vi "Calculate Normals for Mesh.vi"(9 "Color Binding Mode":T1(ring), 10 "Vertex Array":cluster{"X":sgl, "Y":sgl, "Z":sgl}[](array[cluster]), 11 "Draw Mode":T2(ring)) -> (3 "Normal Array":cluster{"X":sgl, "Y":sgl, "Z":sgl}[](array[cluster]))   [LabVIEW 2017, in "NI_3D Picture Control.lvlib"]
uses:
  <vilib>/picture/3D Picture Control/NI_3D Picture Control.lvlib
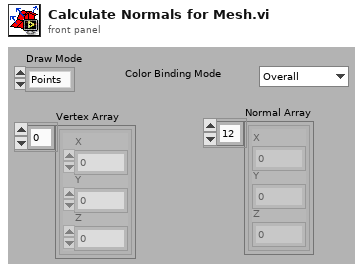
[diagram p1: front panel]
types:
  T1 = enum16{"Overall", "Per Primitive", "Per Vertex", "Binding Off"}
  T2 = enum16{"Points", "Lines", "Line Strip", "Line Loop", "Triangles", "Triangle Strip", "Triangle Fan", "Quads", "Quad Strip", "Polygon"}
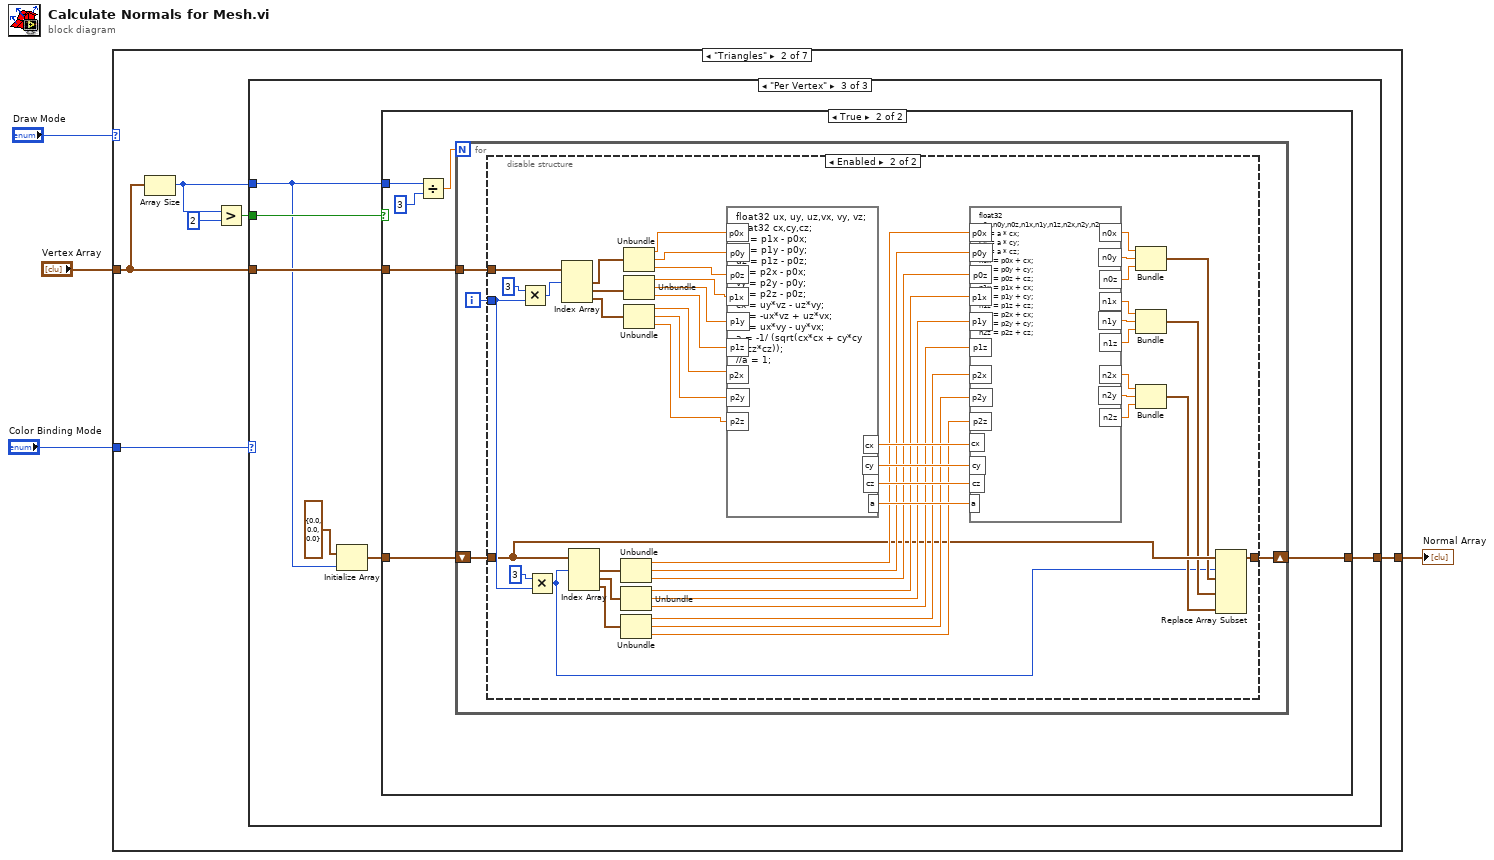
[diagram p0: block diagram]
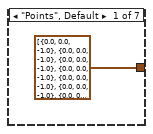
[diagram p2: hidden frame]
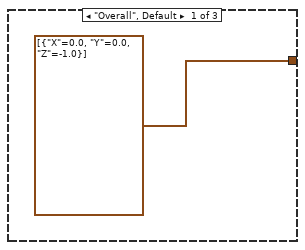
[diagram p3: hidden frame]
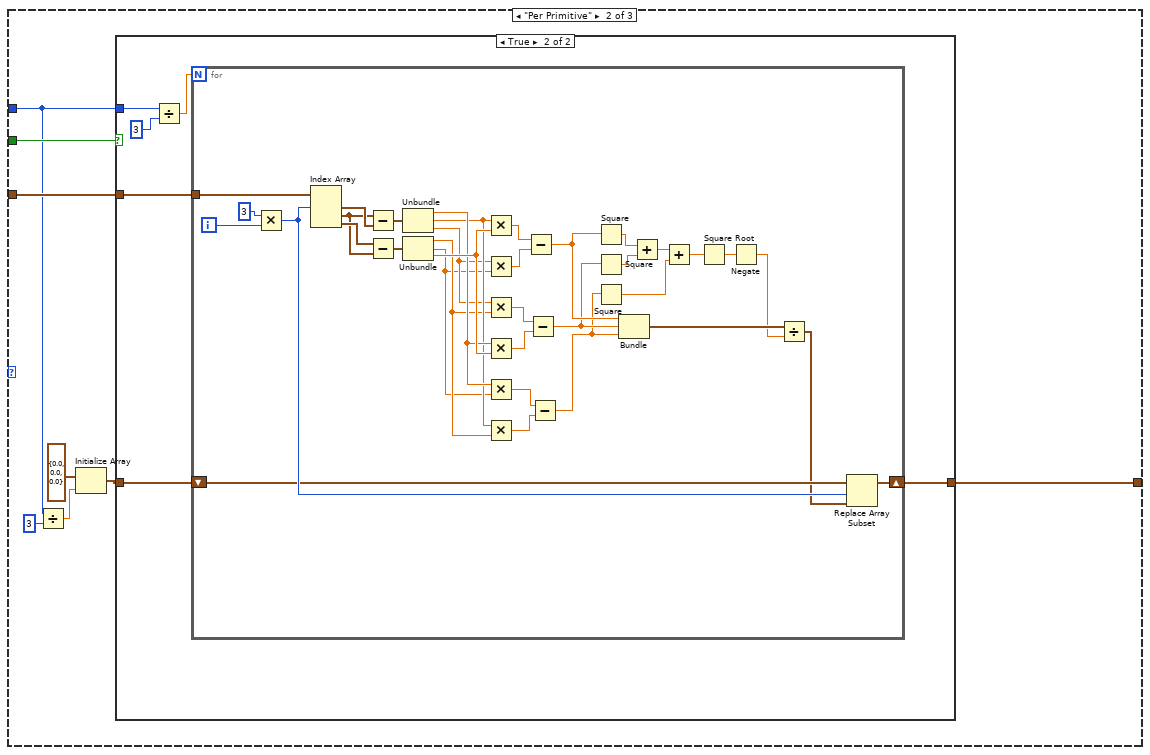
[diagram p4: hidden frame]
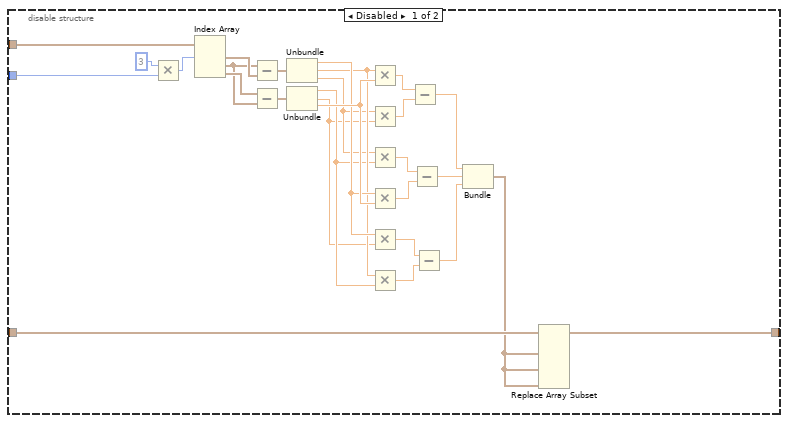
[diagram p7: hidden frame]
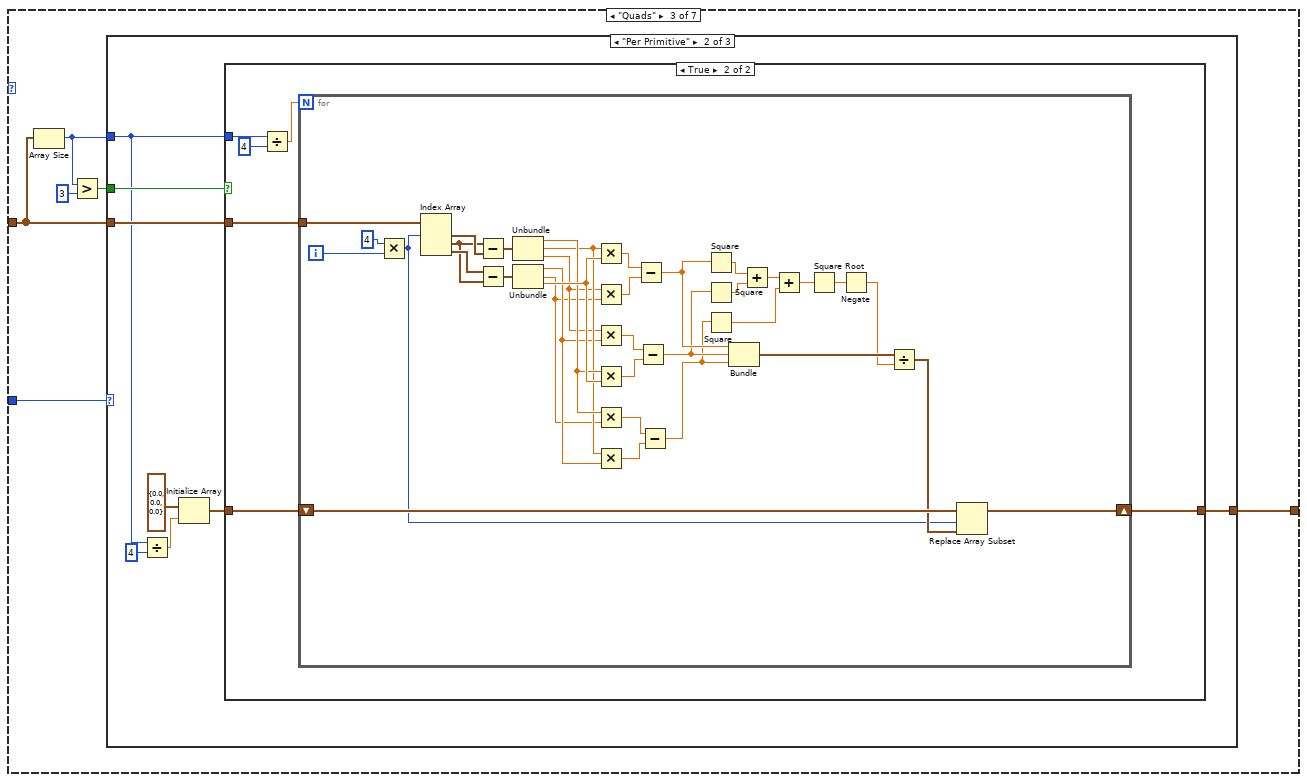
[diagram p8: hidden frame]
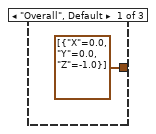
[diagram p9: hidden frame]
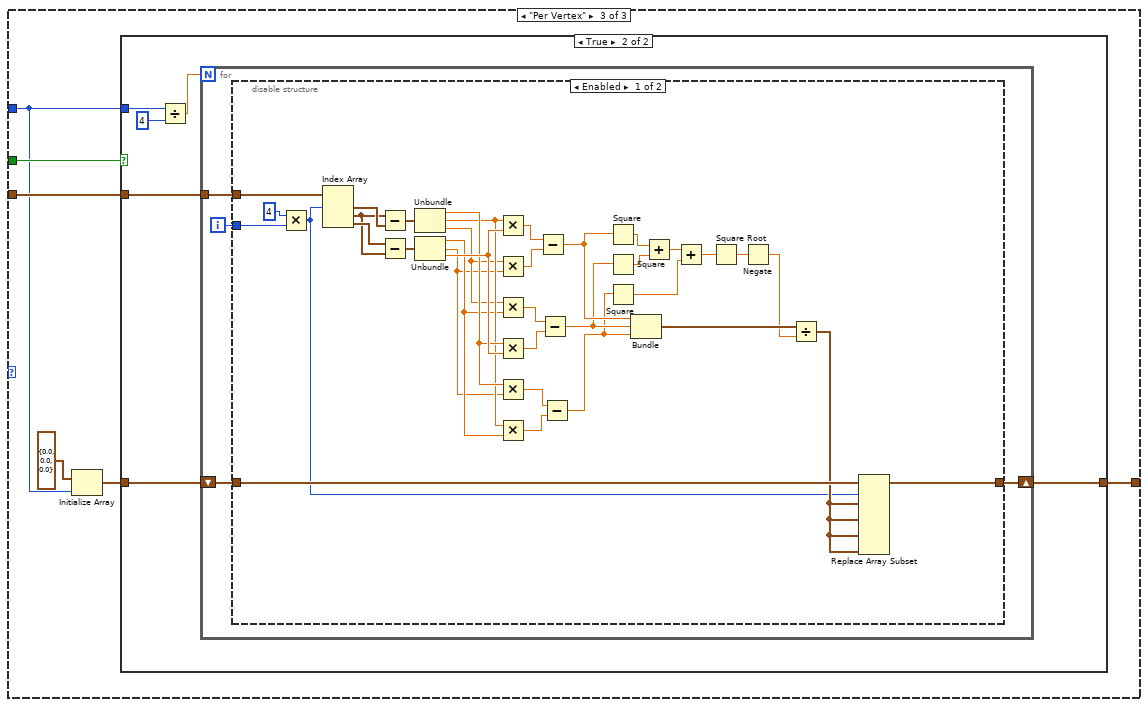
[diagram p11: hidden frame]
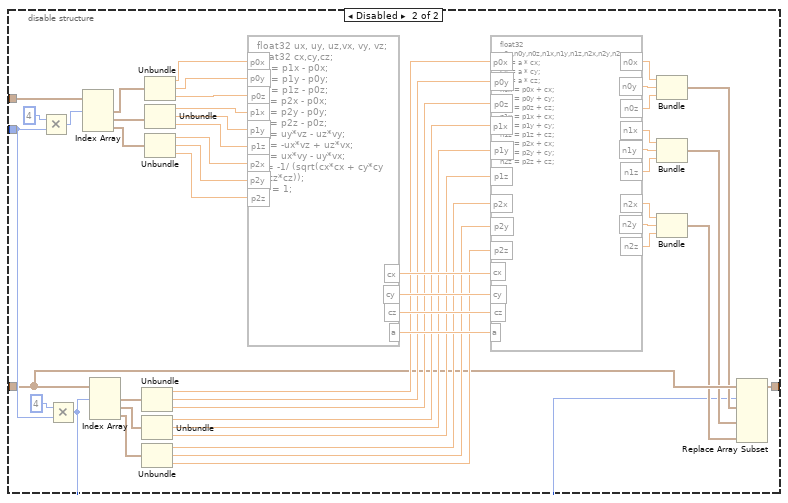
[diagram p13: hidden frame]
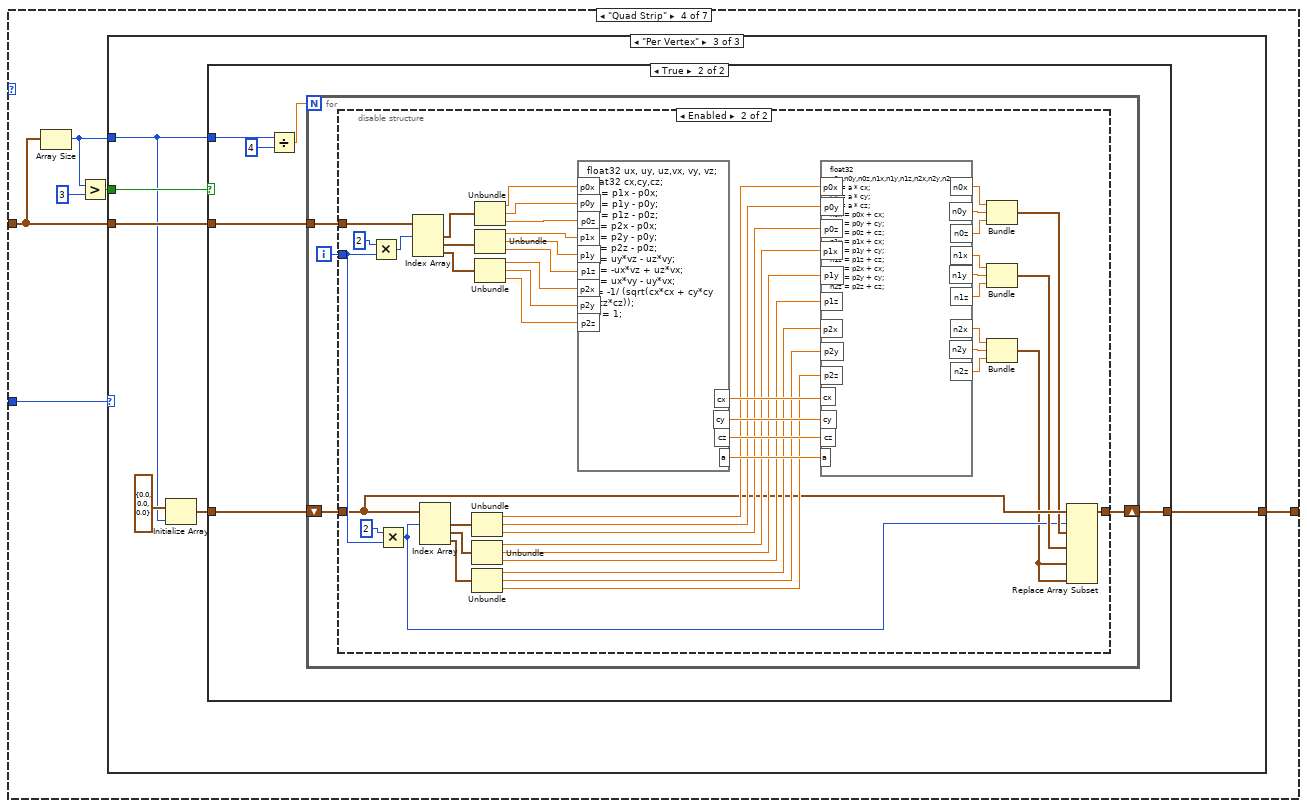
[diagram p14: hidden frame]
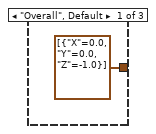
[diagram p15: hidden frame]
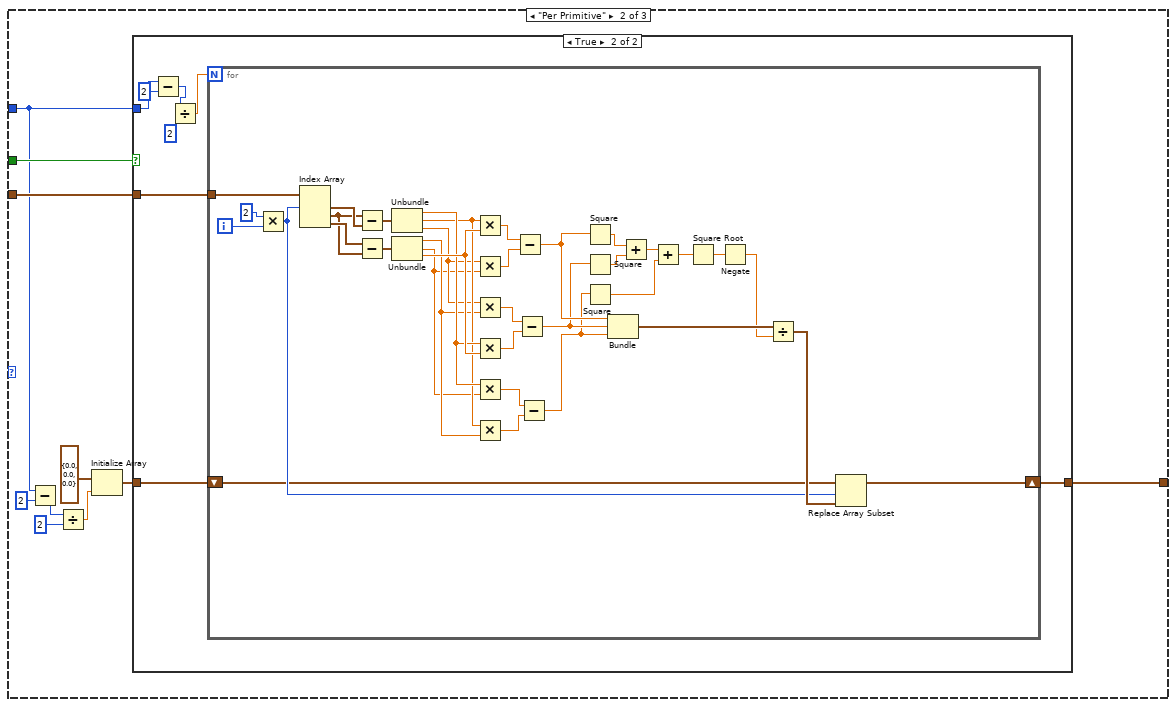
[diagram p16: hidden frame]
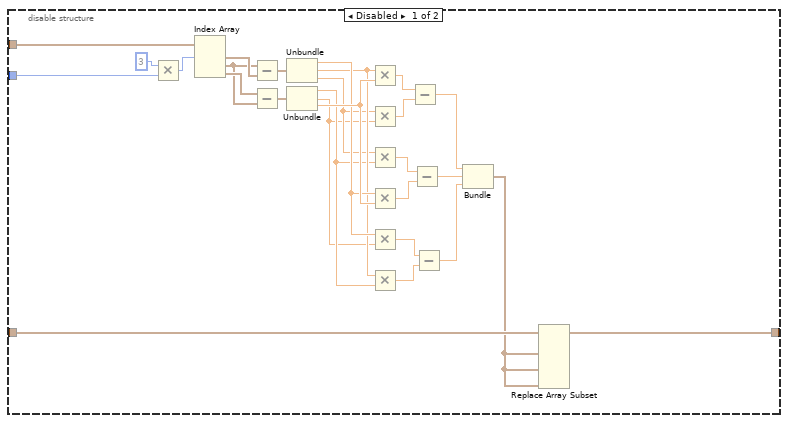
[diagram p19: hidden frame]
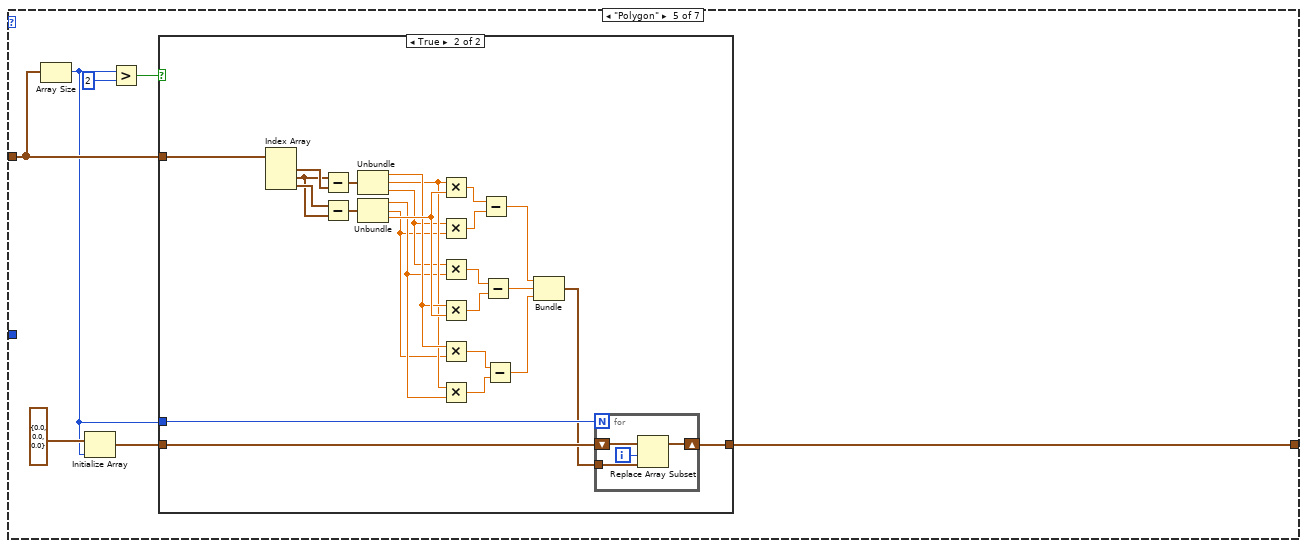
[diagram p20: hidden frame]
diagram:
  n1 = case shown="\"Triangles\"" "Draw Mode" {
    tunnel: "Vertex Array" -> [_ w11 w158 w313 w465 w500 w609]
    tunnel: [cluster{"X":sgl, "Y":sgl, "Z":sgl}[] [{"X"=0.0, "Y"=0.0, "Z"=-1.0}, {"X"=0.0, "Y"=0.0, "Z"=-1.0}, {"X"=0.0, "Y"=0.0, "Z"=-1.0}, {"X"=0.0, "Y"=0.0, "Z"=-1.0}, {"X"=0.0, "Y"=0.0, "Z"=-1.0}, {"X"=0.0, "Y"=0.0, "Z"=-1.0}, {"X"=0.0, "Y"=0.0, "Z"=-1.0}, {"X"=0.0, "Y"=0.0, "Z"=-1.0}, {"X"=0.0, "Y"=0.0, "Z"=-1.0}, {"X"=0.0, "Y"=0.0, "Z"=-1.0}] w10 w157 w312 w459 w499 w608] -> w2
    tunnel: "Color Binding Mode" -> [_ w7 w154 w308 _ w495 w604]
    frame "Points", Default {
    }
    frame "Triangles" {
      n2 = Array Size(array=w11) -> (size(s)=w6:i32)
      n3 = Greater?(x=w6, y=2) -> (0:w8:bool)
      n4 = case shown="\"Per Vertex\"" w7 {
        tunnel: w11 -> [_ w20 w67]
        tunnel: [cluster{"X":sgl, "Y":sgl, "Z":sgl}[] [{"X"=0.0, "Y"=0.0, "Z"=-1.0}] w19 w66] -> w10
        tunnel: w6 -> [_ w13 w62]
        tunnel: w8 -> [_ w18 w65]
        frame "Overall", Default {
        }
        frame "Per Primitive" {
          n5 = Divide(x=w13, y=3) -> (x/y=w15:dbl)
          n6 = Initialize Array(cluster{"X":sgl, "Y":sgl, "Z":sgl} {"X"=0.0, "Y"=0.0, "Z"=0.0} ("element"), w15) -> (w14:cluster{"X":sgl, "Y":sgl, "Z":sgl}[])
          n7 = case shown="True" w18 {
            tunnel: w20 -> [_ w26]
            tunnel: w14 -> [_ w23]
            tunnel: [_ w22] -> w19
            tunnel: w13 -> [_ w21]
            frame False {
            }
            frame True {
              n8 = Divide(x=w21, y=3) -> (x/y=w24:dbl)
              n9 = for {
                N: w24 -> [_]
                tunnel: w26 -> [w31]
                shift-right: [w27] -> w22
                shift-left: w23 -> [w29]
                i -> [w61]
                n10 = Multiply(x=3, y=w61) -> (x*y=w30:i32)
                n11 = Index Array(array=w31, index #1=w30) -> (element #1=w58:cluster{"X":sgl, "Y":sgl, "Z":sgl}, element #2=w57:cluster{"X":sgl, "Y":sgl, "Z":sgl}, element #3=w59:cluster{"X":sgl, "Y":sgl, "Z":sgl})  [unwired: 2 in]
                n12 = Subtract(x=w57, y=w58) -> (x-y=w55:cluster{"X":sgl, "Y":sgl, "Z":sgl})
                n13 = Subtract(x=w59, y=w57) -> (x-y=w56:cluster{"X":sgl, "Y":sgl, "Z":sgl})
                n14 = Unbundle(w55) -> ("X"=w53:sgl, "Y"=w52:sgl, "Z"=w51:sgl)
                n15 = Unbundle(w56) -> ("X"=w50:sgl, "Y"=w49:sgl, "Z"=w54:sgl)
                n16 = Multiply(x=w52, y=w54) -> (x*y=w48:sgl)
                n17 = Multiply(x=w51, y=w49) -> (x*y=w47:sgl)
                n18 = Multiply(x=w51, y=w50) -> (x*y=w45:sgl)
                n19 = Multiply(x=w53, y=w54) -> (x*y=w46:sgl)
                n20 = Multiply(x=w53, y=w49) -> (x*y=w43:sgl)
                n21 = Multiply(x=w52, y=w50) -> (x*y=w44:sgl)
                n22 = Subtract(x=w48, y=w47) -> (x-y=w37:sgl)
                n23 = Subtract(x=w45, y=w46) -> (x-y=w36:sgl)
                n24 = Subtract(x=w43, y=w44) -> (x-y=w35:sgl)
                n25 = Square(x=w37) -> (x^2=w41:sgl)
                n26 = Square(x=w36) -> (x^2=w42:sgl)
                n27 = Square(x=w35) -> (x^2=w39:sgl)
                n28 = Bundle(w37, w36, w35) -> (w34:cluster{sgl, sgl, sgl})  [unwired: 1 in]
                n29 = Add(x=w41, y=w42) -> (x+y=w40:sgl)
                n30 = Add(x=w40, y=w39) -> (x+y=w38:sgl)
                n31 = Square Root(x=w38) -> (sqrt(x)=w33:sgl)
                n32 = Negate(x=w33) -> (-x=w32:sgl)
                n33 = Divide(x=w34, y=w32) -> (x/y=w28:cluster{sgl, sgl, sgl})
                n34 = Replace Array Subset(array=w29, new element=w28, index=w30) -> (w27:cluster{"X":sgl, "Y":sgl, "Z":sgl}[])
              }
            }
          }
        }
        frame "Per Vertex" {
          n35 = Initialize Array(cluster{"X":sgl, "Y":sgl, "Z":sgl} {"X"=0.0, "Y"=0.0, "Z"=0.0} ("element"), w62) -> (w63:cluster{"X":sgl, "Y":sgl, "Z":sgl}[])
          n36 = case shown="True" w65 {
            tunnel: w67 -> [_ w73]
            tunnel: w63 -> [_ w70]
            tunnel: [_ w69] -> w66
            tunnel: w62 -> [_ w68]
            frame False {
            }
            frame True {
              n37 = Divide(x=w68, y=3) -> (x/y=w71:dbl)
              n38 = for {
                N: w71 -> [_]
                tunnel: w73 -> [w77]
                shift-right: [w74] -> w69
                shift-left: w70 -> [w75]
                i -> [w76]
                n39 = disable-structure shown="Enabled" {
                  disable-tunnel: w77 -> [w104 w150]
                  disable-tunnel: w76 -> [w103 w135]
                  disable-tunnel: w75 -> [w80 w109]
                  disable-tunnel: [w79 w110] -> w74
                  frame Disabled {
                    n40 = Multiply(x=3, y=w103) -> (x*y=w101:i32)
                    n41 = Index Array(array=w104, index #1=w101) -> (element #1=w99:cluster{"X":sgl, "Y":sgl, "Z":sgl}, element #2=w98:cluster{"X":sgl, "Y":sgl, "Z":sgl}, element #3=w100:cluster{"X":sgl, "Y":sgl, "Z":sgl})  [unwired: 2 in]
                    n42 = Subtract(x=w98, y=w99) -> (x-y=w96:cluster{"X":sgl, "Y":sgl, "Z":sgl})
                    n43 = Subtract(x=w100, y=w98) -> (x-y=w97:cluster{"X":sgl, "Y":sgl, "Z":sgl})
                    n44 = Unbundle(w96) -> ("X"=w94:sgl, "Y"=w93:sgl, "Z"=w92:sgl)
                    n45 = Unbundle(w97) -> ("X"=w91:sgl, "Y"=w90:sgl, "Z"=w95:sgl)
                    n46 = Multiply(x=w93, y=w95) -> (x*y=w89:sgl)
                    n47 = Multiply(x=w92, y=w90) -> (x*y=w88:sgl)
                    n48 = Multiply(x=w92, y=w91) -> (x*y=w86:sgl)
                    n49 = Multiply(x=w94, y=w95) -> (x*y=w87:sgl)
                    n50 = Multiply(x=w94, y=w90) -> (x*y=w84:sgl)
                    n51 = Multiply(x=w93, y=w91) -> (x*y=w85:sgl)
                    n52 = Subtract(x=w89, y=w88) -> (x-y=w82:sgl)
                    n53 = Subtract(x=w86, y=w87) -> (x-y=w83:sgl)
                    n54 = Subtract(x=w84, y=w85) -> (x-y=w81:sgl)
                    n55 = Bundle(w82, w83, w81) -> (w78:cluster{sgl, sgl, sgl})  [unwired: 1 in]
                    n56 = Replace Array Subset(array=w80, new element #1=w78, new element #2=w78, new element #3=w78) -> (w79:cluster{"X":sgl, "Y":sgl, "Z":sgl}[])  [unwired: 3 in]
                  }
                  frame Enabled {
                    n57 = Multiply(x=3, y=w135) -> (x*y=w151:i32)
                    n58 = Multiply(x=3, y=w135) -> (x*y=w105:i32)
                    n59 = Index Array(array=w150, index #1=w151) -> (element #1=w132:cluster{"X":sgl, "Y":sgl, "Z":sgl}, element #2=w133:cluster{"X":sgl, "Y":sgl, "Z":sgl}, element #3=w134:cluster{"X":sgl, "Y":sgl, "Z":sgl})  [unwired: 2 in]
                    n60 = Index Array(array=w109, index #1=w105) -> (element #1=w122:cluster{"X":sgl, "Y":sgl, "Z":sgl}, element #2=w121:cluster{"X":sgl, "Y":sgl, "Z":sgl}, element #3=w120:cluster{"X":sgl, "Y":sgl, "Z":sgl})  [unwired: 2 in]
                    n61 = Unbundle(w122) -> ("X"=w119:sgl, "Y"=w118:sgl, "Z"=w117:sgl)
                    n62 = Unbundle(w121) -> ("X"=w116:sgl, "Y"=w115:sgl, "Z"=w114:sgl)
                    n63 = Unbundle(w120) -> ("X"=w113:sgl, "Y"=w112:sgl, "Z"=w111:sgl)
                    n64 = Unbundle(w132) -> ("X"=w131:sgl, "Y"=w130:sgl, "Z"=w129:sgl)
                    n65 = Unbundle(w133) -> ("X"=w128:sgl, "Y"=w127:sgl, "Z"=w126:sgl)
                    n66 = Unbundle(w134) -> ("X"=w125:sgl, "Y"=w124:sgl, "Z"=w123:sgl)
                    n67 = formula code="float32 ux, uy, uz,vx, vy, vz; \nfloat32 cx,cy,cz; \nux = p1x - p0x; \nuy = p1y - p0y; \nuz = p1z - p0z; \nvx = p2x - p0x; \nvy = p2y - p0y; \nvz = p2z - p0z; \ncx = uy*vz - uz*vy;\ncy = -ux*vz + uz*vx;\ncz = ux*vy - uy*vx;\na = -1/ (sqrt(cx*cx + cy*cy + cz*cz));\n//a = 1;"("p0x"=w131, "p0y"=w130, "p0z"=w129, "p1x"=w128, "p1y"=w127, "p1z"=w126, "p2x"=w125, "p2y"=w124, "p2z"=w123) -> ("cx"=w139:sgl, "cy"=w138:sgl, "cz"=w137:sgl, "a"=w140:dbl)
                    n68 = formula code="float32 n0x,n0y,n0z,n1x,n1y,n1z,n2x,n2y,n2z;\ncx = a * cx; \ncy = a * cy; \ncz = a * cz; \nn0x = p0x + cx; \nn0y = p0y + cy;\nn0z = p0z + cz;\nn1x = p1x + cx; \nn1y = p1y + cy;\nn1z = p1z + cz;\nn2x = p2x + cx; \nn2y = p2y + cy;\nn2z = p2z + cz;"("p0x"=w119, "p0y"=w118, "p0z"=w117, "p1x"=w116, "p1y"=w115, "p1z"=w114, "p2x"=w113, "p2y"=w112, "p2z"=w111, "cx"=w139, "cy"=w138, "cz"=w137, "a"=w140) -> ("n0x"=w149:sgl, "n0y"=w148:sgl, "n0z"=w147:sgl, "n1x"=w146:sgl, "n1y"=w145:sgl, "n1z"=w144:sgl, "n2x"=w143:sgl, "n2y"=w142:sgl, "n2z"=w141:sgl)
                    n69 = Bundle(w149, w148, w147) -> (w108:cluster{sgl, sgl, sgl})  [unwired: 1 in]
                    n70 = Bundle(w146, w145, w144) -> (w107:cluster{sgl, sgl, sgl})  [unwired: 1 in]
                    n71 = Bundle(w143, w142, w141) -> (w106:cluster{sgl, sgl, sgl})  [unwired: 1 in]
                    n72 = Replace Array Subset(array=w109, new element #1=w108, index #1=w105, new element #2=w107, new element #3=w106) -> (w110:cluster{"X":sgl, "Y":sgl, "Z":sgl}[])  [unwired: 2 in]
                  }
                }
              }
            }
          }
        }
      }
    }
    frame "Quads" {
      n73 = Array Size(array=w158) -> (size(s)=w153:i32)
      n74 = Greater?(x=w153, y=3) -> (0:w155:bool)
      n75 = case shown="\"Per Primitive\"" w154 {
        tunnel: w158 -> [_ w167 w214]
        tunnel: [cluster{"X":sgl, "Y":sgl, "Z":sgl}[] [{"X"=0.0, "Y"=0.0, "Z"=-1.0}] w166 w213] -> w157
        tunnel: w153 -> [_ w160 w210]
        tunnel: w155 -> [_ w165 w212]
        frame "Overall", Default {
        }
        frame "Per Primitive" {
          n76 = Divide(x=w160, y=4) -> (x/y=w162:dbl)
          n77 = Initialize Array(cluster{"X":sgl, "Y":sgl, "Z":sgl} {"X"=0.0, "Y"=0.0, "Z"=0.0} ("element"), w162) -> (w161:cluster{"X":sgl, "Y":sgl, "Z":sgl}[])
          n78 = case shown="True" w165 {
            tunnel: w167 -> [_ w171]
            tunnel: w161 -> [_ w169]
            tunnel: [_ w168] -> w166
            tunnel: w160 -> [_ w172]
            frame False {
            }
            frame True {
              n79 = Divide(x=w172, y=4) -> (x/y=w170:dbl)
              n80 = for {
                N: w170 -> [_]
                tunnel: w171 -> [w208]
                shift-right: [w205] -> w168
                shift-left: w169 -> [w206]
                i -> [w207]
                n81 = Multiply(x=4, y=w207) -> (x*y=w175:i32)
                n82 = Index Array(array=w208, index #1=w175) -> (element #1=w202:cluster{"X":sgl, "Y":sgl, "Z":sgl}, element #2=w201:cluster{"X":sgl, "Y":sgl, "Z":sgl}, element #3=w203:cluster{"X":sgl, "Y":sgl, "Z":sgl})  [unwired: 2 in]
                n83 = Subtract(x=w201, y=w202) -> (x-y=w199:cluster{"X":sgl, "Y":sgl, "Z":sgl})
                n84 = Subtract(x=w203, y=w201) -> (x-y=w200:cluster{"X":sgl, "Y":sgl, "Z":sgl})
                n85 = Unbundle(w199) -> ("X"=w197:sgl, "Y"=w196:sgl, "Z"=w195:sgl)
                n86 = Unbundle(w200) -> ("X"=w194:sgl, "Y"=w193:sgl, "Z"=w198:sgl)
                n87 = Multiply(x=w196, y=w198) -> (x*y=w192:sgl)
                n88 = Multiply(x=w195, y=w193) -> (x*y=w191:sgl)
                n89 = Multiply(x=w195, y=w194) -> (x*y=w189:sgl)
                n90 = Multiply(x=w197, y=w198) -> (x*y=w190:sgl)
                n91 = Multiply(x=w197, y=w193) -> (x*y=w187:sgl)
                n92 = Multiply(x=w196, y=w194) -> (x*y=w188:sgl)
                n93 = Subtract(x=w192, y=w191) -> (x-y=w181:sgl)
                n94 = Subtract(x=w189, y=w190) -> (x-y=w180:sgl)
                n95 = Subtract(x=w187, y=w188) -> (x-y=w179:sgl)
                n96 = Square(x=w181) -> (x^2=w185:sgl)
                n97 = Square(x=w180) -> (x^2=w186:sgl)
                n98 = Square(x=w179) -> (x^2=w183:sgl)
                n99 = Bundle(w181, w180, w179) -> (w178:cluster{sgl, sgl, sgl})  [unwired: 1 in]
                n100 = Add(x=w185, y=w186) -> (x+y=w184:sgl)
                n101 = Add(x=w184, y=w183) -> (x+y=w182:sgl)
                n102 = Square Root(x=w182) -> (sqrt(x)=w177:sgl)
                n103 = Negate(x=w177) -> (-x=w174:sgl)
                n104 = Divide(x=w178, y=w174) -> (x/y=w176:cluster{sgl, sgl, sgl})
                n105 = Replace Array Subset(array=w206, new element=w176, index=w175) -> (w205:cluster{"X":sgl, "Y":sgl, "Z":sgl}[])
              }
            }
          }
        }
        frame "Per Vertex" {
          n106 = Initialize Array(cluster{"X":sgl, "Y":sgl, "Z":sgl} {"X"=0.0, "Y"=0.0, "Z"=0.0} ("element"), w210) -> (w209:cluster{"X":sgl, "Y":sgl, "Z":sgl}[])
          n107 = case shown="True" w212 {
            tunnel: w214 -> [_ w218]
            tunnel: w209 -> [_ w216]
            tunnel: [_ w215] -> w213
            tunnel: w210 -> [_ w219]
            frame False {
            }
            frame True {
              n108 = Divide(x=w219, y=4) -> (x/y=w217:dbl)
              n109 = for {
                N: w217 -> [_]
                tunnel: w218 -> [w224]
                shift-right: [w221] -> w215
                shift-left: w216 -> [w222]
                i -> [w223]
                n110 = disable-structure shown="Enabled" {
                  disable-tunnel: w224 -> [w259 w305]
                  disable-tunnel: w223 -> [w258 w290]
                  disable-tunnel: w222 -> [w239 w264]
                  disable-tunnel: [w238 w265] -> w221
                  frame Enabled {
                    n111 = Multiply(x=4, y=w258) -> (x*y=w226:i32)
                    n112 = Index Array(array=w259, index #1=w226) -> (element #1=w255:cluster{"X":sgl, "Y":sgl, "Z":sgl}, element #2=w254:cluster{"X":sgl, "Y":sgl, "Z":sgl}, element #3=w256:cluster{"X":sgl, "Y":sgl, "Z":sgl})  [unwired: 2 in]
                    n113 = Subtract(x=w254, y=w255) -> (x-y=w252:cluster{"X":sgl, "Y":sgl, "Z":sgl})
                    n114 = Subtract(x=w256, y=w254) -> (x-y=w253:cluster{"X":sgl, "Y":sgl, "Z":sgl})
                    n115 = Unbundle(w252) -> ("X"=w250:sgl, "Y"=w249:sgl, "Z"=w248:sgl)
                    n116 = Unbundle(w253) -> ("X"=w247:sgl, "Y"=w246:sgl, "Z"=w251:sgl)
                    n117 = Multiply(x=w249, y=w251) -> (x*y=w245:sgl)
                    n118 = Multiply(x=w248, y=w246) -> (x*y=w244:sgl)
                    n119 = Multiply(x=w248, y=w247) -> (x*y=w242:sgl)
                    n120 = Multiply(x=w250, y=w251) -> (x*y=w243:sgl)
                    n121 = Multiply(x=w250, y=w246) -> (x*y=w240:sgl)
                    n122 = Multiply(x=w249, y=w247) -> (x*y=w241:sgl)
                    n123 = Subtract(x=w245, y=w244) -> (x-y=w232:sgl)
                    n124 = Subtract(x=w242, y=w243) -> (x-y=w231:sgl)
                    n125 = Subtract(x=w240, y=w241) -> (x-y=w230:sgl)
                    n126 = Square(x=w232) -> (x^2=w236:sgl)
                    n127 = Square(x=w231) -> (x^2=w237:sgl)
                    n128 = Square(x=w230) -> (x^2=w234:sgl)
                    n129 = Bundle(w232, w231, w230) -> (w229:cluster{sgl, sgl, sgl})  [unwired: 1 in]
                    n130 = Add(x=w236, y=w237) -> (x+y=w235:sgl)
                    n131 = Add(x=w235, y=w234) -> (x+y=w233:sgl)
                    n132 = Square Root(x=w233) -> (sqrt(x)=w228:sgl)
                    n133 = Negate(x=w228) -> (-x=w225:sgl)
                    n134 = Divide(x=w229, y=w225) -> (x/y=w227:cluster{sgl, sgl, sgl})
                    n135 = Replace Array Subset(array=w239, new element #1=w227, index #1=w226, new element #2=w227, new element #3=w227, new element #4=w227) -> (w238:cluster{"X":sgl, "Y":sgl, "Z":sgl}[])  [unwired: 3 in]
                  }
                  frame Disabled {
                    n136 = Multiply(x=4, y=w290) -> (x*y=w306:i32)
                    n137 = Multiply(x=4, y=w290) -> (x*y=w260:i32)
                    n138 = Index Array(array=w305, index #1=w306) -> (element #1=w287:cluster{"X":sgl, "Y":sgl, "Z":sgl}, element #2=w288:cluster{"X":sgl, "Y":sgl, "Z":sgl}, element #3=w289:cluster{"X":sgl, "Y":sgl, "Z":sgl})  [unwired: 2 in]
                    n139 = Index Array(array=w264, index #1=w260) -> (element #1=w277:cluster{"X":sgl, "Y":sgl, "Z":sgl}, element #2=w276:cluster{"X":sgl, "Y":sgl, "Z":sgl}, element #3=w275:cluster{"X":sgl, "Y":sgl, "Z":sgl})  [unwired: 2 in]
                    n140 = Unbundle(w277) -> ("X"=w274:sgl, "Y"=w273:sgl, "Z"=w272:sgl)
                    n141 = Unbundle(w276) -> ("X"=w271:sgl, "Y"=w270:sgl, "Z"=w269:sgl)
                    n142 = Unbundle(w275) -> ("X"=w268:sgl, "Y"=w267:sgl, "Z"=w266:sgl)
                    n143 = Unbundle(w287) -> ("X"=w286:sgl, "Y"=w285:sgl, "Z"=w284:sgl)
                    n144 = Unbundle(w288) -> ("X"=w283:sgl, "Y"=w282:sgl, "Z"=w281:sgl)
                    n145 = Unbundle(w289) -> ("X"=w280:sgl, "Y"=w279:sgl, "Z"=w278:sgl)
                    n146 = formula code="float32 ux, uy, uz,vx, vy, vz; \nfloat32 cx,cy,cz; \nux = p1x - p0x; \nuy = p1y - p0y; \nuz = p1z - p0z; \nvx = p2x - p0x; \nvy = p2y - p0y; \nvz = p2z - p0z; \ncx = uy*vz - uz*vy;\ncy = -ux*vz + uz*vx;\ncz = ux*vy - uy*vx;\na = -1/ (sqrt(cx*cx + cy*cy + cz*cz));\n//a = 1;"("p0x"=w286, "p0y"=w285, "p0z"=w284, "p1x"=w283, "p1y"=w282, "p1z"=w281, "p2x"=w280, "p2y"=w279, "p2z"=w278) -> ("cx"=w294:sgl, "cy"=w293:sgl, "cz"=w292:sgl, "a"=w295:dbl)
                    n147 = formula code="float32 n0x,n0y,n0z,n1x,n1y,n1z,n2x,n2y,n2z;\ncx = a * cx; \ncy = a * cy; \ncz = a * cz; \nn0x = p0x + cx; \nn0y = p0y + cy;\nn0z = p0z + cz;\nn1x = p1x + cx; \nn1y = p1y + cy;\nn1z = p1z + cz;\nn2x = p2x + cx; \nn2y = p2y + cy;\nn2z = p2z + cz;"("p0x"=w274, "p0y"=w273, "p0z"=w272, "p1x"=w271, "p1y"=w270, "p1z"=w269, "p2x"=w268, "p2y"=w267, "p2z"=w266, "cx"=w294, "cy"=w293, "cz"=w292, "a"=w295) -> ("n0x"=w304:sgl, "n0y"=w303:sgl, "n0z"=w302:sgl, "n1x"=w301:sgl, "n1y"=w300:sgl, "n1z"=w299:sgl, "n2x"=w298:sgl, "n2y"=w297:sgl, "n2z"=w296:sgl)
                    n148 = Bundle(w304, w303, w302) -> (w263:cluster{sgl, sgl, sgl})  [unwired: 1 in]
                    n149 = Bundle(w301, w300, w299) -> (w262:cluster{sgl, sgl, sgl})  [unwired: 1 in]
                    n150 = Bundle(w298, w297, w296) -> (w261:cluster{sgl, sgl, sgl})  [unwired: 1 in]
                    n151 = Replace Array Subset(array=w264, new element #1=w263, index #1=w260, new element #2=w262, new element #3=w261) -> (w265:cluster{"X":sgl, "Y":sgl, "Z":sgl}[])  [unwired: 2 in]
                  }
                }
              }
            }
          }
        }
      }
    }
    frame "Quad Strip" {
      n152 = Array Size(array=w313) -> (size(s)=w311:i32)
      n153 = Greater?(x=w311, y=3) -> (0:w309:bool)
      n154 = case shown="\"Per Vertex\"" w308 {
        tunnel: w313 -> [_ w324 w373]
        tunnel: [cluster{"X":sgl, "Y":sgl, "Z":sgl}[] [{"X"=0.0, "Y"=0.0, "Z"=-1.0}] w323 w372] -> w312
        tunnel: w311 -> [_ w316 w368]
        tunnel: w309 -> [_ w322 w371]
        frame "Overall", Default {
        }
        frame "Per Primitive" {
          n155 = Subtract(x=w316, y=2) -> (x-y=w315:i32)
          n156 = Divide(x=w315, y=2) -> (x/y=w318:dbl)
          n157 = Initialize Array(cluster{"X":sgl, "Y":sgl, "Z":sgl} {"X"=0.0, "Y"=0.0, "Z"=0.0} ("element"), w318) -> (w320:cluster{"X":sgl, "Y":sgl, "Z":sgl}[])
          n158 = case shown="True" w322 {
            tunnel: w324 -> [_ w331]
            tunnel: w320 -> [_ w329]
            tunnel: [_ w328] -> w323
            tunnel: w316 -> [_ w326]
            frame False {
            }
            frame True {
              n159 = Subtract(x=w326, y=2) -> (x-y=w325:i32)
              n160 = Divide(x=w325, y=2) -> (x/y=w330:dbl)
              n161 = for {
                N: w330 -> [_]
                tunnel: w331 -> [w336]
                shift-right: [w333] -> w328
                shift-left: w329 -> [w334]
                i -> [w335]
                n162 = Multiply(x=2, y=w335) -> (x*y=w338:i32)
                n163 = Index Array(array=w336, index #1=w338) -> (element #1=w365:cluster{"X":sgl, "Y":sgl, "Z":sgl}, element #2=w364:cluster{"X":sgl, "Y":sgl, "Z":sgl}, element #3=w366:cluster{"X":sgl, "Y":sgl, "Z":sgl})  [unwired: 2 in]
                n164 = Subtract(x=w364, y=w365) -> (x-y=w362:cluster{"X":sgl, "Y":sgl, "Z":sgl})
                n165 = Subtract(x=w366, y=w364) -> (x-y=w363:cluster{"X":sgl, "Y":sgl, "Z":sgl})
                n166 = Unbundle(w362) -> ("X"=w360:sgl, "Y"=w359:sgl, "Z"=w358:sgl)
                n167 = Unbundle(w363) -> ("X"=w357:sgl, "Y"=w356:sgl, "Z"=w361:sgl)
                n168 = Multiply(x=w359, y=w361) -> (x*y=w355:sgl)
                n169 = Multiply(x=w358, y=w356) -> (x*y=w354:sgl)
                n170 = Multiply(x=w358, y=w357) -> (x*y=w352:sgl)
                n171 = Multiply(x=w360, y=w361) -> (x*y=w353:sgl)
                n172 = Multiply(x=w360, y=w356) -> (x*y=w350:sgl)
                n173 = Multiply(x=w359, y=w357) -> (x*y=w351:sgl)
                n174 = Subtract(x=w355, y=w354) -> (x-y=w344:sgl)
                n175 = Subtract(x=w352, y=w353) -> (x-y=w343:sgl)
                n176 = Subtract(x=w350, y=w351) -> (x-y=w342:sgl)
                n177 = Square(x=w344) -> (x^2=w348:sgl)
                n178 = Square(x=w343) -> (x^2=w349:sgl)
                n179 = Square(x=w342) -> (x^2=w346:sgl)
                n180 = Bundle(w344, w343, w342) -> (w341:cluster{sgl, sgl, sgl})  [unwired: 1 in]
                n181 = Add(x=w348, y=w349) -> (x+y=w347:sgl)
                n182 = Add(x=w347, y=w346) -> (x+y=w345:sgl)
                n183 = Square Root(x=w345) -> (sqrt(x)=w340:sgl)
                n184 = Negate(x=w340) -> (-x=w337:sgl)
                n185 = Divide(x=w341, y=w337) -> (x/y=w339:cluster{sgl, sgl, sgl})
                n186 = Replace Array Subset(array=w334, new element=w339, index=w338) -> (w333:cluster{"X":sgl, "Y":sgl, "Z":sgl}[])
              }
            }
          }
        }
        frame "Per Vertex" {
          n187 = Initialize Array(cluster{"X":sgl, "Y":sgl, "Z":sgl} {"X"=0.0, "Y"=0.0, "Z"=0.0} ("element"), w368) -> (w369:cluster{"X":sgl, "Y":sgl, "Z":sgl}[])
          n188 = case shown="True" w371 {
            tunnel: w373 -> [_ w377]
            tunnel: w369 -> [_ w375]
            tunnel: [_ w374] -> w372
            tunnel: w368 -> [_ w378]
            frame False {
            }
            frame True {
              n189 = Divide(x=w378, y=4) -> (x/y=w376:dbl)
              n190 = for {
                N: w376 -> [_]
                tunnel: w377 -> [w383]
                shift-right: [w380] -> w374
                shift-left: w375 -> [w381]
                i -> [w382]
                n191 = disable-structure shown="Enabled" {
                  disable-tunnel: w383 -> [w410 w456]
                  disable-tunnel: w382 -> [w409 w441]
                  disable-tunnel: w381 -> [w386 w415]
                  disable-tunnel: [w385 w416] -> w380
                  frame Disabled {
                    n192 = Multiply(x=3, y=w409) -> (x*y=w407:i32)
                    n193 = Index Array(array=w410, index #1=w407) -> (element #1=w405:cluster{"X":sgl, "Y":sgl, "Z":sgl}, element #2=w404:cluster{"X":sgl, "Y":sgl, "Z":sgl}, element #3=w406:cluster{"X":sgl, "Y":sgl, "Z":sgl})  [unwired: 2 in]
                    n194 = Subtract(x=w404, y=w405) -> (x-y=w402:cluster{"X":sgl, "Y":sgl, "Z":sgl})
                    n195 = Subtract(x=w406, y=w404) -> (x-y=w403:cluster{"X":sgl, "Y":sgl, "Z":sgl})
                    n196 = Unbundle(w402) -> ("X"=w400:sgl, "Y"=w399:sgl, "Z"=w398:sgl)
                    n197 = Unbundle(w403) -> ("X"=w397:sgl, "Y"=w396:sgl, "Z"=w401:sgl)
                    n198 = Multiply(x=w399, y=w401) -> (x*y=w395:sgl)
                    n199 = Multiply(x=w398, y=w396) -> (x*y=w394:sgl)
                    n200 = Multiply(x=w398, y=w397) -> (x*y=w392:sgl)
                    n201 = Multiply(x=w400, y=w401) -> (x*y=w393:sgl)
                    n202 = Multiply(x=w400, y=w396) -> (x*y=w390:sgl)
                    n203 = Multiply(x=w399, y=w397) -> (x*y=w391:sgl)
                    n204 = Subtract(x=w395, y=w394) -> (x-y=w388:sgl)
                    n205 = Subtract(x=w392, y=w393) -> (x-y=w389:sgl)
                    n206 = Subtract(x=w390, y=w391) -> (x-y=w387:sgl)
                    n207 = Bundle(w388, w389, w387) -> (w384:cluster{sgl, sgl, sgl})  [unwired: 1 in]
                    n208 = Replace Array Subset(array=w386, new element #1=w384, new element #2=w384, new element #3=w384) -> (w385:cluster{"X":sgl, "Y":sgl, "Z":sgl}[])  [unwired: 3 in]
                  }
                  frame Enabled {
                    n209 = Multiply(x=2, y=w441) -> (x*y=w457:i32)
                    n210 = Multiply(x=2, y=w441) -> (x*y=w412:i32)
                    n211 = Index Array(array=w456, index #1=w457) -> (element #1=w438:cluster{"X":sgl, "Y":sgl, "Z":sgl}, element #2=w439:cluster{"X":sgl, "Y":sgl, "Z":sgl}, element #3=w440:cluster{"X":sgl, "Y":sgl, "Z":sgl})  [unwired: 2 in]
                    n212 = Index Array(array=w415, index #1=w412) -> (element #1=w428:cluster{"X":sgl, "Y":sgl, "Z":sgl}, element #2=w427:cluster{"X":sgl, "Y":sgl, "Z":sgl}, element #3=w426:cluster{"X":sgl, "Y":sgl, "Z":sgl})  [unwired: 2 in]
                    n213 = Unbundle(w428) -> ("X"=w425:sgl, "Y"=w424:sgl, "Z"=w423:sgl)
                    n214 = Unbundle(w427) -> ("X"=w422:sgl, "Y"=w421:sgl, "Z"=w420:sgl)
                    n215 = Unbundle(w426) -> ("X"=w419:sgl, "Y"=w418:sgl, "Z"=w417:sgl)
                    n216 = Unbundle(w438) -> ("X"=w437:sgl, "Y"=w436:sgl, "Z"=w435:sgl)
                    n217 = Unbundle(w439) -> ("X"=w434:sgl, "Y"=w433:sgl, "Z"=w432:sgl)
                    n218 = Unbundle(w440) -> ("X"=w431:sgl, "Y"=w430:sgl, "Z"=w429:sgl)
                    n219 = formula code="float32 ux, uy, uz,vx, vy, vz; \nfloat32 cx,cy,cz; \nux = p1x - p0x; \nuy = p1y - p0y; \nuz = p1z - p0z; \nvx = p2x - p0x; \nvy = p2y - p0y; \nvz = p2z - p0z; \ncx = uy*vz - uz*vy;\ncy = -ux*vz + uz*vx;\ncz = ux*vy - uy*vx;\na = -1/ (sqrt(cx*cx + cy*cy + cz*cz));\n//a = 1;"("p0x"=w437, "p0y"=w436, "p0z"=w435, "p1x"=w434, "p1y"=w433, "p1z"=w432, "p2x"=w431, "p2y"=w430, "p2z"=w429) -> ("cx"=w445:sgl, "cy"=w444:sgl, "cz"=w443:sgl, "a"=w446:dbl)
                    n220 = formula code="float32 n0x,n0y,n0z,n1x,n1y,n1z,n2x,n2y,n2z;\ncx = a * cx; \ncy = a * cy; \ncz = a * cz; \nn0x = p0x + cx; \nn0y = p0y + cy;\nn0z = p0z + cz;\nn1x = p1x + cx; \nn1y = p1y + cy;\nn1z = p1z + cz;\nn2x = p2x + cx; \nn2y = p2y + cy;\nn2z = p2z + cz;"("p0x"=w425, "p0y"=w424, "p0z"=w423, "p1x"=w422, "p1y"=w421, "p1z"=w420, "p2x"=w419, "p2y"=w418, "p2z"=w417, "cx"=w445, "cy"=w444, "cz"=w443, "a"=w446) -> ("n0x"=w455:sgl, "n0y"=w454:sgl, "n0z"=w453:sgl, "n1x"=w452:sgl, "n1y"=w451:sgl, "n1z"=w450:sgl, "n2x"=w449:sgl, "n2y"=w448:sgl, "n2z"=w447:sgl)
                    n221 = Bundle(w455, w454, w453) -> (w414:cluster{sgl, sgl, sgl})  [unwired: 1 in]
                    n222 = Bundle(w452, w451, w450) -> (w413:cluster{sgl, sgl, sgl})  [unwired: 1 in]
                    n223 = Bundle(w449, w448, w447) -> (w411:cluster{sgl, sgl, sgl})  [unwired: 1 in]
                    n224 = Replace Array Subset(array=w415, new element #1=w414, index #1=w412, new element #2=w413, new element #3=w411, new element #4=w411) -> (w416:cluster{"X":sgl, "Y":sgl, "Z":sgl}[])  [unwired: 3 in]
                  }
                }
              }
            }
          }
        }
      }
    }
    frame "Polygon" {
      n225 = Array Size(array=w465) -> (size(s)=w460:i32)
      n226 = Initialize Array(cluster{"X":sgl, "Y":sgl, "Z":sgl} {"X"=0.0, "Y"=0.0, "Z"=0.0} ("element"), w460) -> (w463:cluster{"X":sgl, "Y":sgl, "Z":sgl}[])
      n227 = Greater?(x=w460, y=2) -> (0:w461:bool)
      n228 = case shown="True" w461 {
        tunnel: w465 -> [_ w490]
        tunnel: w463 -> [_ w468]
        tunnel: w460 -> [_ w469]
        tunnel: [_ w466] -> w459
        frame False {
        }
        frame True {
          n229 = Index Array(array=w490) -> (element #1=w488:cluster{"X":sgl, "Y":sgl, "Z":sgl}, element #2=w487:cluster{"X":sgl, "Y":sgl, "Z":sgl}, element #3=w489:cluster{"X":sgl, "Y":sgl, "Z":sgl})  [unwired: 3 in]
          n230 = Subtract(x=w487, y=w488) -> (x-y=w485:cluster{"X":sgl, "Y":sgl, "Z":sgl})
          n231 = Subtract(x=w489, y=w487) -> (x-y=w486:cluster{"X":sgl, "Y":sgl, "Z":sgl})
          n232 = Unbundle(w485) -> ("X"=w483:sgl, "Y"=w482:sgl, "Z"=w481:sgl)
          n233 = Unbundle(w486) -> ("X"=w480:sgl, "Y"=w479:sgl, "Z"=w484:sgl)
          n234 = Multiply(x=w482, y=w484) -> (x*y=w478:sgl)
          n235 = Multiply(x=w481, y=w479) -> (x*y=w477:sgl)
          n236 = Multiply(x=w481, y=w480) -> (x*y=w475:sgl)
          n237 = Multiply(x=w483, y=w484) -> (x*y=w476:sgl)
          n238 = Multiply(x=w483, y=w479) -> (x*y=w473:sgl)
          n239 = Multiply(x=w482, y=w480) -> (x*y=w474:sgl)
          n240 = Subtract(x=w478, y=w477) -> (x-y=w471:sgl)
          n241 = Subtract(x=w475, y=w476) -> (x-y=w472:sgl)
          n242 = Subtract(x=w473, y=w474) -> (x-y=w470:sgl)
          n243 = Bundle(w471, w472, w470) -> (w467:cluster{sgl, sgl, sgl})  [unwired: 1 in]
          n244 = for {
            N: w469 -> [_]
            shift-right: [w491] -> w466
            shift-left: w468 -> [w494]
            tunnel: w467 -> [w492]
            i -> [w493]
            n245 = Replace Array Subset(array=w494, new element=w492, index=w493) -> (w491:cluster{"X":sgl, "Y":sgl, "Z":sgl}[])
          }
        }
      }
    }
    frame "Triangle Strip" {
      n246 = Array Size(array=w500) -> (size(s)=w496:i32)
      n247 = Greater?(x=w496, y=2) -> (0:w497:bool)
      n248 = case shown="\"Per Vertex\"" w495 {
        tunnel: w500 -> [_ w509 w553]
        tunnel: [cluster{"X":sgl, "Y":sgl, "Z":sgl}[] [{"X"=0.0, "Y"=0.0, "Z"=-1.0}] w508 w552] -> w499
        tunnel: w497 -> [_ w507 w551]
        tunnel: w496 -> [_ w502 w548]
        frame "Overall", Default {
        }
        frame "Per Primitive" {
          n249 = Subtract(x=w502, y=2) -> (x-y=w503:i32)
          n250 = Initialize Array(cluster{"X":sgl, "Y":sgl, "Z":sgl} {"X"=0.0, "Y"=0.0, "Z"=0.0} ("element"), w503) -> (w505:cluster{"X":sgl, "Y":sgl, "Z":sgl}[])
          n251 = case shown="True" w507 {
            tunnel: w509 -> [_ w515]
            tunnel: w505 -> [_ w514]
            tunnel: [_ w513] -> w508
            tunnel: w502 -> [_ w512]
            frame False {
            }
            frame True {
              n252 = Subtract(x=w512, y=2) -> (x-y=w511:i32)
              n253 = for {
                N: w511 -> [_]
                tunnel: w515 -> [w520]
                shift-right: [w518] -> w513
                shift-left: w514 -> [w519]
                i -> [w517]
                n254 = Index Array(array=w520, index #1=w517) -> (element #1=w546:cluster{"X":sgl, "Y":sgl, "Z":sgl}, element #2=w545:cluster{"X":sgl, "Y":sgl, "Z":sgl}, element #3=w547:cluster{"X":sgl, "Y":sgl, "Z":sgl})  [unwired: 2 in]
                n255 = Subtract(x=w545, y=w546) -> (x-y=w543:cluster{"X":sgl, "Y":sgl, "Z":sgl})
                n256 = Subtract(x=w547, y=w545) -> (x-y=w544:cluster{"X":sgl, "Y":sgl, "Z":sgl})
                n257 = Unbundle(w543) -> ("X"=w541:sgl, "Y"=w540:sgl, "Z"=w539:sgl)
                n258 = Unbundle(w544) -> ("X"=w538:sgl, "Y"=w537:sgl, "Z"=w542:sgl)
                n259 = Multiply(x=w540, y=w542) -> (x*y=w536:sgl)
                n260 = Multiply(x=w539, y=w537) -> (x*y=w535:sgl)
                n261 = Multiply(x=w539, y=w538) -> (x*y=w533:sgl)
                n262 = Multiply(x=w541, y=w542) -> (x*y=w534:sgl)
                n263 = Multiply(x=w541, y=w537) -> (x*y=w531:sgl)
                n264 = Multiply(x=w540, y=w538) -> (x*y=w532:sgl)
                n265 = Subtract(x=w536, y=w535) -> (x-y=w525:sgl)
                n266 = Subtract(x=w533, y=w534) -> (x-y=w524:sgl)
                n267 = Subtract(x=w531, y=w532) -> (x-y=w523:sgl)
                n268 = Square(x=w525) -> (x^2=w529:sgl)
                n269 = Square(x=w524) -> (x^2=w530:sgl)
                n270 = Square(x=w523) -> (x^2=w527:sgl)
                n271 = Bundle(w525, w524, w523) -> (w522:cluster{sgl, sgl, sgl})  [unwired: 1 in]
                n272 = Add(x=w529, y=w530) -> (x+y=w528:sgl)
                n273 = Add(x=w528, y=w527) -> (x+y=w526:sgl)
                n274 = Square Root(x=w526) -> (sqrt(x)=w516:sgl)
                n275 = Divide(x=w522, y=w516) -> (x/y=w521:cluster{sgl, sgl, sgl})
                n276 = Replace Array Subset(array=w519, new element=w521, index=w517) -> (w518:cluster{"X":sgl, "Y":sgl, "Z":sgl}[])
              }
            }
          }
        }
        frame "Per Vertex" {
          n277 = Initialize Array(cluster{"X":sgl, "Y":sgl, "Z":sgl} {"X"=0.0, "Y"=0.0, "Z"=0.0} ("element"), w548) -> (w549:cluster{"X":sgl, "Y":sgl, "Z":sgl}[])
          n278 = case shown="True" w551 {
            tunnel: w553 -> [_ w559]
            tunnel: w549 -> [_ w558]
            tunnel: [_ w557] -> w552
            tunnel: w548 -> [_ w556]
            frame False {
            }
            frame True {
              n279 = Subtract(x=w556, y=2) -> (x-y=w555:i32)
              n280 = for {
                N: w555 -> [_]
                tunnel: w559 -> [w603]
                shift-right: [w601] -> w557
                shift-left: w558 -> [w602]
                i -> [w600]
                n281 = Index Array(array=w603, index #1=w600) -> (element #1=w585:cluster{"X":sgl, "Y":sgl, "Z":sgl}, element #2=w586:cluster{"X":sgl, "Y":sgl, "Z":sgl}, element #3=w584:cluster{"X":sgl, "Y":sgl, "Z":sgl})  [unwired: 2 in]
                n282 = Index Array(array=w602, index #1=w600) -> (element #1=w583:cluster{"X":sgl, "Y":sgl, "Z":sgl}, element #2=w582:cluster{"X":sgl, "Y":sgl, "Z":sgl}, element #3=w581:cluster{"X":sgl, "Y":sgl, "Z":sgl})  [unwired: 2 in]
                n283 = Unbundle(w585) -> ("X"=w580:sgl, "Y"=w579:sgl, "Z"=w578:sgl)
                n284 = Unbundle(w586) -> ("X"=w577:sgl, "Y"=w576:sgl, "Z"=w575:sgl)
                n285 = Unbundle(w584) -> ("X"=w574:sgl, "Y"=w573:sgl, "Z"=w572:sgl)
                n286 = Unbundle(w583) -> ("X"=w571:sgl, "Y"=w570:sgl, "Z"=w569:sgl)
                n287 = Unbundle(w582) -> ("X"=w568:sgl, "Y"=w567:sgl, "Z"=w566:sgl)
                n288 = Unbundle(w581) -> ("X"=w565:sgl, "Y"=w564:sgl, "Z"=w563:sgl)
                n289 = formula code="float32 ux, uy, uz,vx, vy, vz; \nfloat32 cx,cy,cz; \nux = p1x - p0x; \nuy = p1y - p0y; \nuz = p1z - p0z; \nvx = p2x - p0x; \nvy = p2y - p0y; \nvz = p2z - p0z; \ncx = uy*vz - uz*vy;\ncy = -ux*vz + uz*vx;\ncz = ux*vy - uy*vx;\na = -1/ (sqrt(cx*cx + cy*cy + cz*cz));\n//a = 1;"("p0x"=w580, "p0y"=w579, "p0z"=w578, "p1x"=w577, "p1y"=w576, "p1z"=w575, "p2x"=w574, "p2y"=w573, "p2z"=w572) -> ("cx"=w589:sgl, "cy"=w588:sgl, "cz"=w587:sgl, "a"=w590:dbl)
                n290 = formula code="float32 n0x,n0y,n0z,n1x,n1y,n1z,n2x,n2y,n2z;\ncx = a * cx; \ncy = a * cy; \ncz = a * cz; \nn0x = p0x + cx; \nn0y = p0y + cy;\nn0z = p0z + cz;\nn1x = p1x + cx; \nn1y = p1y + cy;\nn1z = p1z + cz;\nn2x = p2x + cx; \nn2y = p2y + cy;\nn2z = p2z + cz;"("p0x"=w571, "p0y"=w570, "p0z"=w569, "p1x"=w568, "p1y"=w567, "p1z"=w566, "p2x"=w565, "p2y"=w564, "p2z"=w563, "cx"=w589, "cy"=w588, "cz"=w587, "a"=w590) -> ("n0x"=w599:sgl, "n0y"=w598:sgl, "n0z"=w597:sgl, "n1x"=w596:sgl, "n1y"=w595:sgl, "n1z"=w594:sgl, "n2x"=w593:sgl, "n2y"=w592:sgl, "n2z"=w591:sgl)
                n291 = Bundle(w599, w598, w597) -> (w562:cluster{sgl, sgl, sgl})  [unwired: 1 in]
                n292 = Bundle(w596, w595, w594) -> (w561:cluster{sgl, sgl, sgl})  [unwired: 1 in]
                n293 = Bundle(w593, w592, w591) -> (w560:cluster{sgl, sgl, sgl})  [unwired: 1 in]
                n294 = Replace Array Subset(array=w602, new element #1=w562, index #1=w600, new element #2=w561, new element #3=w560) -> (w601:cluster{"X":sgl, "Y":sgl, "Z":sgl}[])  [unwired: 2 in]
              }
            }
          }
        }
      }
    }
    frame "Triangle Fan" {
      n295 = Array Size(array=w609) -> (size(s)=w605:i32)
      n296 = Greater?(x=w605, y=2) -> (0:w606:bool)
      n297 = case shown="\"Per Primitive\"" w604 {
        tunnel: w609 -> [_ w618 w663]
        tunnel: [cluster{"X":sgl, "Y":sgl, "Z":sgl}[] [{"X"=0.0, "Y"=0.0, "Z"=-1.0}] w617 w662] -> w608
        tunnel: w606 -> [_ w616 w661]
        tunnel: w605 -> [_ w611 w658]
        frame "Overall", Default {
        }
        frame "Per Primitive" {
          n298 = Subtract(x=w611, y=2) -> (x-y=w612:i32)
          n299 = Initialize Array(cluster{"X":sgl, "Y":sgl, "Z":sgl} {"X"=0.0, "Y"=0.0, "Z"=0.0} ("element"), w612) -> (w614:cluster{"X":sgl, "Y":sgl, "Z":sgl}[])
          n300 = case shown="True" w616 {
            tunnel: w618 -> [_ w624]
            tunnel: w614 -> [_ w623]
            tunnel: [_ w622] -> w617
            tunnel: w611 -> [_ w621]
            frame False {
            }
            frame True {
              n301 = Subtract(x=w621, y=2) -> (x-y=w619:i32)
              n302 = for {
                N: w619 -> [_]
                tunnel: w624 -> [w628]
                shift-right: [w626] -> w622
                shift-left: w623 -> [w627]
                i -> [w625]
                n303 = Index Array(array=w628, index #2=w625) -> (element #1=w656:cluster{"X":sgl, "Y":sgl, "Z":sgl}, element #2=w655:cluster{"X":sgl, "Y":sgl, "Z":sgl}, element #3=w657:cluster{"X":sgl, "Y":sgl, "Z":sgl})  [unwired: 2 in]
                n304 = Subtract(x=w655, y=w656) -> (x-y=w653:cluster{"X":sgl, "Y":sgl, "Z":sgl})
                n305 = Subtract(x=w657, y=w655) -> (x-y=w654:cluster{"X":sgl, "Y":sgl, "Z":sgl})
                n306 = Unbundle(w653) -> ("X"=w651:sgl, "Y"=w650:sgl, "Z"=w649:sgl)
                n307 = Unbundle(w654) -> ("X"=w648:sgl, "Y"=w647:sgl, "Z"=w652:sgl)
                n308 = Multiply(x=w650, y=w652) -> (x*y=w646:sgl)
                n309 = Multiply(x=w649, y=w647) -> (x*y=w645:sgl)
                n310 = Multiply(x=w649, y=w648) -> (x*y=w643:sgl)
                n311 = Multiply(x=w651, y=w652) -> (x*y=w644:sgl)
                n312 = Multiply(x=w651, y=w647) -> (x*y=w641:sgl)
                n313 = Multiply(x=w650, y=w648) -> (x*y=w642:sgl)
                n314 = Subtract(x=w646, y=w645) -> (x-y=w635:sgl)
                n315 = Subtract(x=w643, y=w644) -> (x-y=w634:sgl)
                n316 = Subtract(x=w641, y=w642) -> (x-y=w633:sgl)
                n317 = Square(x=w635) -> (x^2=w639:sgl)
                n318 = Square(x=w634) -> (x^2=w640:sgl)
                n319 = Square(x=w633) -> (x^2=w637:sgl)
                n320 = Bundle(w635, w634, w633) -> (w632:cluster{sgl, sgl, sgl})  [unwired: 1 in]
                n321 = Add(x=w639, y=w640) -> (x+y=w638:sgl)
                n322 = Add(x=w638, y=w637) -> (x+y=w636:sgl)
                n323 = Square Root(x=w636) -> (sqrt(x)=w631:sgl)
                n324 = Negate(x=w631) -> (-x=w629:sgl)
                n325 = Divide(x=w632, y=w629) -> (x/y=w630:cluster{sgl, sgl, sgl})
                n326 = Replace Array Subset(array=w627, new element=w630, index=w625) -> (w626:cluster{"X":sgl, "Y":sgl, "Z":sgl}[])
              }
            }
          }
        }
        frame "Per Vertex" {
          n327 = Initialize Array(cluster{"X":sgl, "Y":sgl, "Z":sgl} {"X"=0.0, "Y"=0.0, "Z"=0.0} ("element"), w658) -> (w659:cluster{"X":sgl, "Y":sgl, "Z":sgl}[])
          n328 = case shown="True" w661 {
            tunnel: w663 -> [_ w669]
            tunnel: w659 -> [_ w668]
            tunnel: [_ w667] -> w662
            tunnel: w658 -> [_ w666]
            frame False {
            }
            frame True {
              n329 = Subtract(x=w666, y=2) -> (x-y=w664:i32)
              n330 = for {
                N: w664 -> [_]
                tunnel: w669 -> [w719]
                shift-right: [w717] -> w667
                shift-left: w668 -> [w718]
                i -> [w716]
                n331 = Increment(x=w716) -> (x+1=w701:i32)
                n332 = Increment(x=w716) -> (x+1=w700:i32)
                n333 = Index Array(array=w719, index #1=0 ("index"), index #2=w701) -> (element #1=w697:cluster{"X":sgl, "Y":sgl, "Z":sgl}, element #2=w698:cluster{"X":sgl, "Y":sgl, "Z":sgl}, element #3=w696:cluster{"X":sgl, "Y":sgl, "Z":sgl})  [unwired: 1 in]
                n334 = Index Array(array=w718, index #1=0 ("index"), index #2=w700) -> (element #1=w695:cluster{"X":sgl, "Y":sgl, "Z":sgl}, element #2=w694:cluster{"X":sgl, "Y":sgl, "Z":sgl}, element #3=w693:cluster{"X":sgl, "Y":sgl, "Z":sgl})  [unwired: 1 in]
                n335 = Unbundle(w697) -> ("X"=w692:sgl, "Y"=w691:sgl, "Z"=w690:sgl)
                n336 = Unbundle(w698) -> ("X"=w689:sgl, "Y"=w688:sgl, "Z"=w687:sgl)
                n337 = Unbundle(w696) -> ("X"=w686:sgl, "Y"=w685:sgl, "Z"=w684:sgl)
                n338 = Unbundle(w695) -> ("X"=w683:sgl, "Y"=w682:sgl, "Z"=w681:sgl)
                n339 = Unbundle(w694) -> ("X"=w680:sgl, "Y"=w679:sgl, "Z"=w678:sgl)
                n340 = Unbundle(w693) -> ("X"=w677:sgl, "Y"=w676:sgl, "Z"=w675:sgl)
                n341 = formula code="float32 ux, uy, uz,vx, vy, vz; \nfloat32 cx,cy,cz; \nux = p1x - p0x; \nuy = p1y - p0y; \nuz = p1z - p0z; \nvx = p2x - p0x; \nvy = p2y - p0y; \nvz = p2z - p0z; \ncx = uy*vz - uz*vy;\ncy = -ux*vz + uz*vx;\ncz = ux*vy - uy*vx;\na = -1/ (sqrt(cx*cx + cy*cy + cz*cz));\n//a = 1;"("p0x"=w692, "p0y"=w691, "p0z"=w690, "p1x"=w689, "p1y"=w688, "p1z"=w687, "p2x"=w686, "p2y"=w685, "p2z"=w684) -> ("cx"=w705:sgl, "cy"=w704:sgl, "cz"=w703:sgl, "a"=w706:dbl)
                n342 = formula code="float32 n0x,n0y,n0z,n1x,n1y,n1z,n2x,n2y,n2z;\ncx = a * cx; \ncy = a * cy; \ncz = a * cz; \nn0x = p0x + cx; \nn0y = p0y + cy;\nn0z = p0z + cz;\nn1x = p1x + cx; \nn1y = p1y + cy;\nn1z = p1z + cz;\nn2x = p2x + cx; \nn2y = p2y + cy;\nn2z = p2z + cz;"("p0x"=w683, "p0y"=w682, "p0z"=w681, "p1x"=w680, "p1y"=w679, "p1z"=w678, "p2x"=w677, "p2y"=w676, "p2z"=w675, "cx"=w705, "cy"=w704, "cz"=w703, "a"=w706) -> ("n0x"=w715:sgl, "n0y"=w714:sgl, "n0z"=w713:sgl, "n1x"=w712:sgl, "n1y"=w711:sgl, "n1z"=w710:sgl, "n2x"=w709:sgl, "n2y"=w708:sgl, "n2z"=w707:sgl)
                n343 = Bundle(w715, w714, w713) -> (w674:cluster{sgl, sgl, sgl})  [unwired: 1 in]
                n344 = Bundle(w712, w711, w710) -> (w673:cluster{sgl, sgl, sgl})  [unwired: 1 in]
                n345 = Bundle(w709, w708, w707) -> (w672:cluster{sgl, sgl, sgl})  [unwired: 1 in]
                n346 = Increment(x=w716) -> (x+1=w670:i32)
                n347 = Replace Array Subset(array=w718, new element #1=w674, index #1=0 ("index"), new element #2=w673, index #2=w670, new element #3=w672) -> (w717:cluster{"X":sgl, "Y":sgl, "Z":sgl}[])  [unwired: 1 in]
              }
            }
          }
        }
      }
    }
  }
  "Normal Array" <- w2
